vi "ApplyCutAndMakeHistogram (SubVI).vi"(0 "Array in":dbl[][](array[numeric]), 5 "Intensity cut":dbl=230.0, 7 "max":dbl=5000.0 format="%#_13g", 9 "min":dbl=1300.0 format="%#_13g", 11 "# bins":i32=370) -> (4 "Array out":dbl[][](array[numeric]), 6 "Histogram Graph":T1)   [LabVIEW 2016]
uses:
  <vilib>/Analysis/NI_AALPro.lvlib
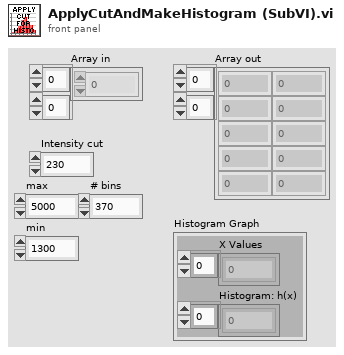
[diagram p1: front panel]
types:
  T1 = cluster{"X Values":dbl[], "Histogram: h(x)":i32[]}
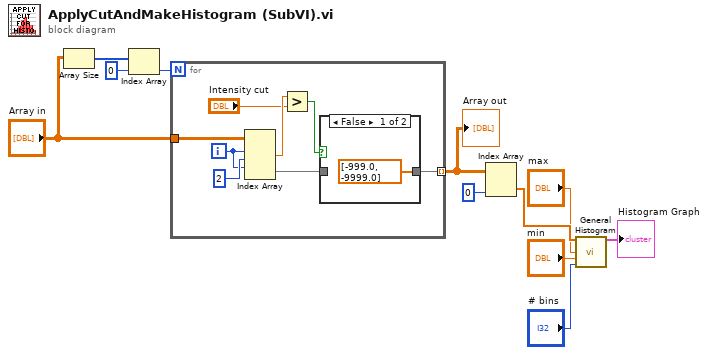
[diagram p0: block diagram]
diagram:
  n1 = Array Size(array="Array in") -> (size(s)=w2:i32[])
  n2 = Index Array(array=w2, index=0) -> (element=w4:i32)
  n3 = for {
    N: w4 -> [_]
    tunnel: "Array in" -> [w19]
    tunnel: [w12] -> w9 mode=indexing
    i -> [w14]
    n4 = Index Array(array=w19, index (row) #1=w14, index (col) #1=2 ("index (row)"), index (row) #2=w14) -> (element #1=w18:dbl, element #2=w13:dbl[])  [unwired: 1 in]
    n5 = Greater?(x=w18, y="Intensity cut") -> (0:w16:bool)
    n6 = case shown="False" w16 {
      tunnel: w13 -> [_ w21]
      tunnel: [dbl[] [-999.0, -9999.0] ("Array") w21] -> w12
      frame False {
      }
      frame True {
      }
    }
  }
  "Array out" <- w9
  n7 = Index Array(array=w9, index (col)=0 ("disabled index (col)")) -> (element=w11:dbl[])  [unwired: 1 in]
  n8 = call <vilib>:"General Histogram.vi"("X"=w11, "max"="max", "min"="min", "# bins"="# bins") -> ("Histogram Graph"=→"Histogram Graph":T1)  [unwired: 7 in, 4 out]
